vi "LEBITplc.CreateSpecialArray.vi"(4 "DBArray":string[][](array[string])) -> (1 "ListOfSpecials":string[](array[string]))   [LabVIEW 2012, in "LEBITplc.lvlib"]
uses:
  LEBITplc.lvlib
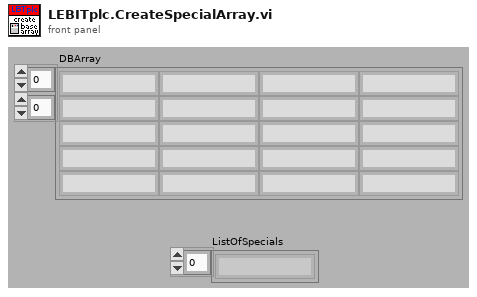
[diagram p1: front panel]
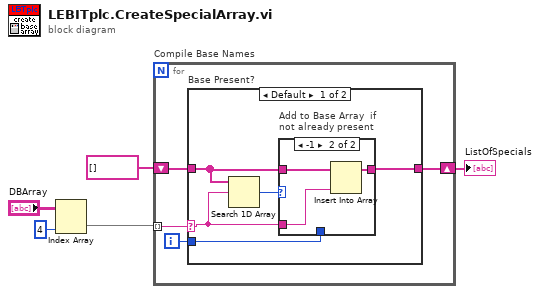
[diagram p0: block diagram]
diagram:
  n1 = Index Array(array="DBArray", index (col)=4 ("disabled index (col)")) -> (element=w2:string[])  [unwired: 1 in]
  n2 = for "Compile Base Names" {
    tunnel: w2 -> [w9] mode=indexing
    shift-right: [w7] -> w1
    shift-left: string[] [] -> [w8]
    i -> [w6]
    n3 = case "Base Present?" shown="Default" w9 {
      selector: w9 -> [w12 _]
      tunnel: w8 -> [w13 w19]
      tunnel: [w11 w19] -> w7
      tunnel: w6 -> [w10 _]
      frame Default {
        n4 = Search 1D Array(1D array=w13, element=w12) -> (index of element=w14:i32)  [unwired: 1 in]
        n5 = case "Add to Base Array  if \nnot already present" shown="-1" w14 {
          tunnel: w13 -> [w15 w18]
          tunnel: w12 -> [_ w16]
          tunnel: [w15 w17] -> w11
          tunnel: w10 -> [_ _]
          frame 0, Default {
          }
          frame -1 {
            n6 = Insert Into Array(array=w18, new element=w16) -> (w17:string[])  [unwired: 1 in]
          }
        }
      }
      frame "" {
      }
    }
  }
  "ListOfSpecials" <- w1
